vi "_SerialCOMTest.vi"() -> ()   [LabVIEW 2020]
uses:
  Processors.ctl
panel:
  out "Version":string
  in  "Python version":string="3.9"
  out "Port":string
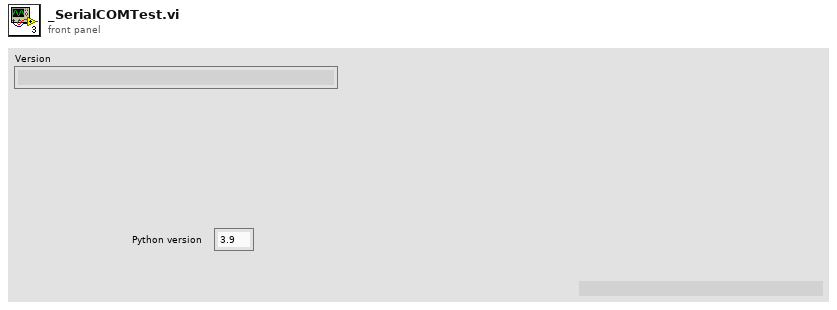
[diagram p1: front panel]
types:
  T1 = typedef "Processors.ctl" = enum16{"SPIKE", "Pi", "Pi_ssh", "OpenMV", "Dunio"}
  T2 = typedef "PythonCtrl.ctl" = cluster{"session":refnum<k35>, "PyPath":path, "Processor":T1, "Port":string, "version":string}
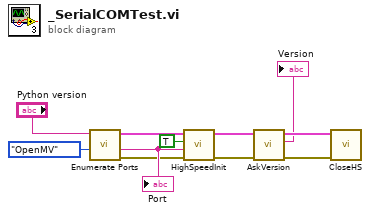
[diagram p0: block diagram]
diagram:
  n1 = call "Enumerate Ports.vi"("Processor"=Processors."OpenMV", "Python version"="Python version") -> ("error out"=w2:errorcluster, "guess"=w6:string, "Python"=w7:T2)  [unwired: 5 in, 2 out]
  "Port" <- w6
  n2 = call "HighSpeedInit.vi"("error in"=w2, "Port"=w6, "Fast"=TRUE, "Python"=w7) -> ("error out"=w9:errorcluster, "Python"=w8:T2)  [unwired: 6 in]
  n3 = call "AskVersion.vi"("error in"=w9, "Python"=w8) -> ("error out"=w5:errorcluster, "Version"=→"Version":string, "Python"=w4:T2)  [unwired: 7 in]
  n4 = call "CloseHS.vi"("error in (no error)"=w5, "Python"=w4) -> ()  [unwired: 10 in]
